vi "ROI_Selection_Limit.vi"(8 "error in (no error)":errorcluster, 9 "ROI in":T1, 10 "Square":bool, 11 "Picture":i32[][](array[numeric])) -> (0 "error out":errorcluster, 1 "ROI out":T1)   [LabVIEW 2011]
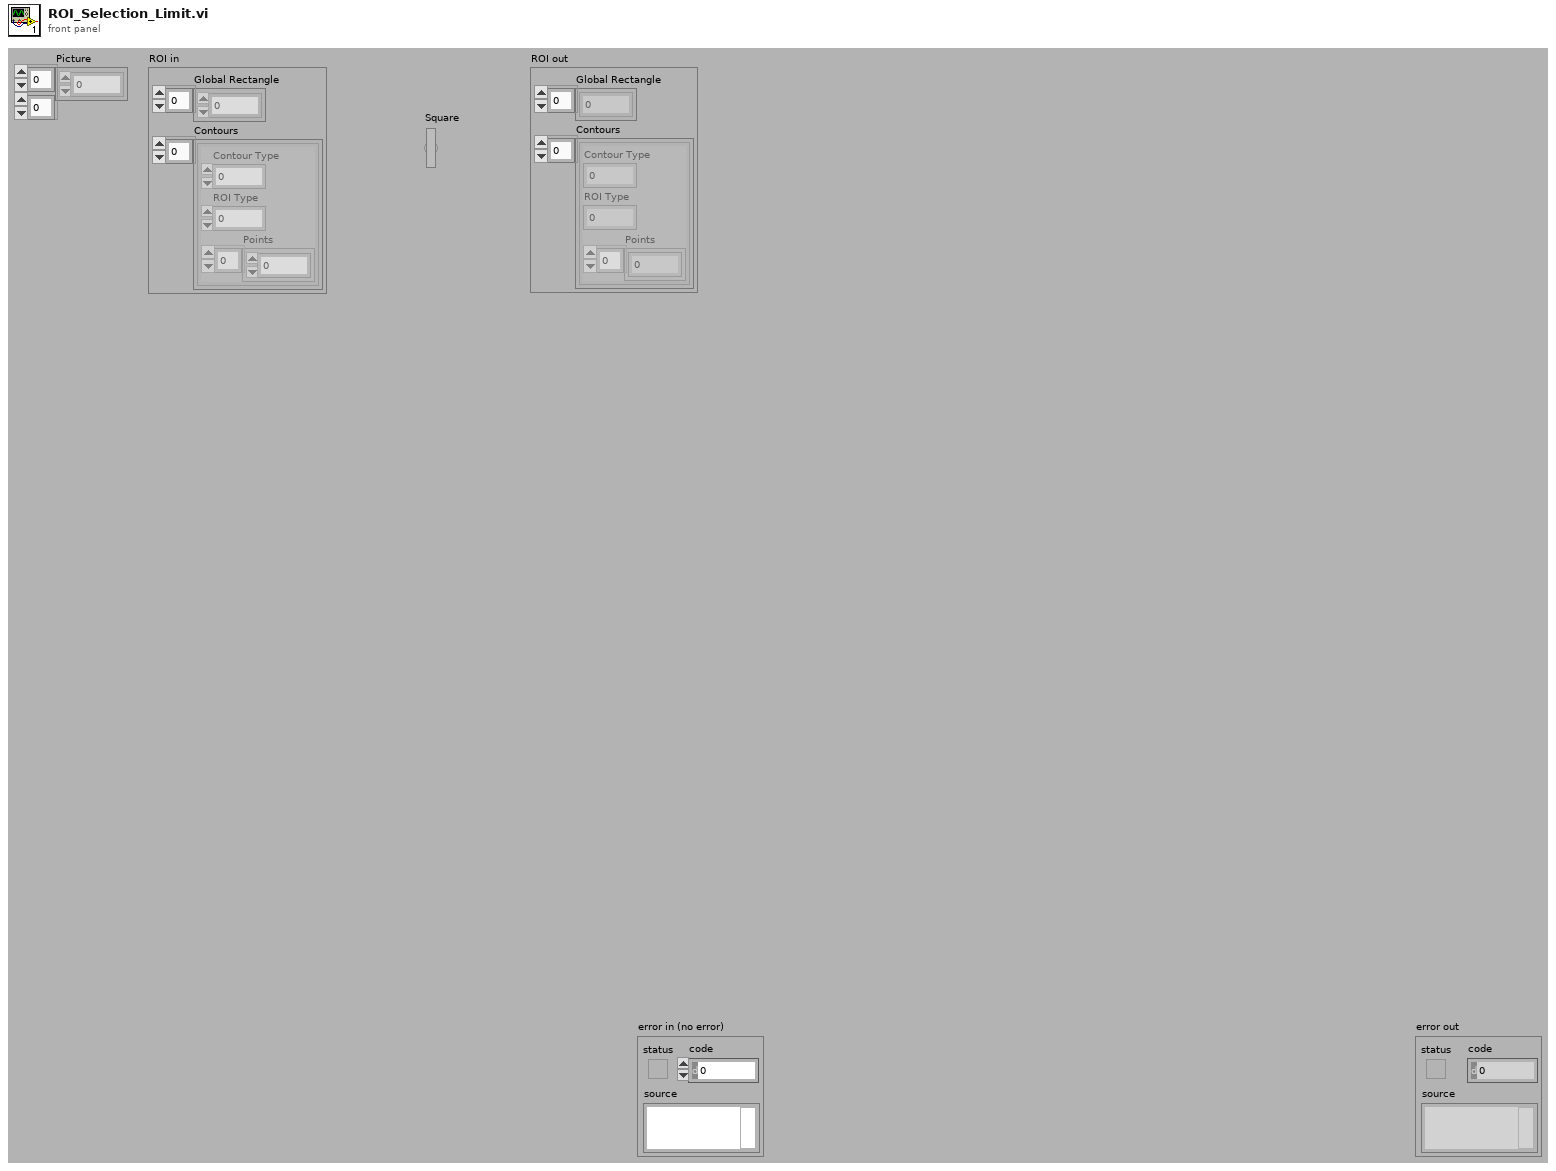
[diagram p1: front panel]
types:
  T1 = cluster{"Global Rectangle":i32[], "Contours":cluster{"Contour Type":u32, "ROI Type":u32, "Points":i32[]}[]}
  T2 = cluster{"Contour Type":u32, "ROI Type":u32, "Points":i32[]}[]
  T3 = cluster{"Contour Type":u32, "ROI Type":u32, "Points":i32[]}
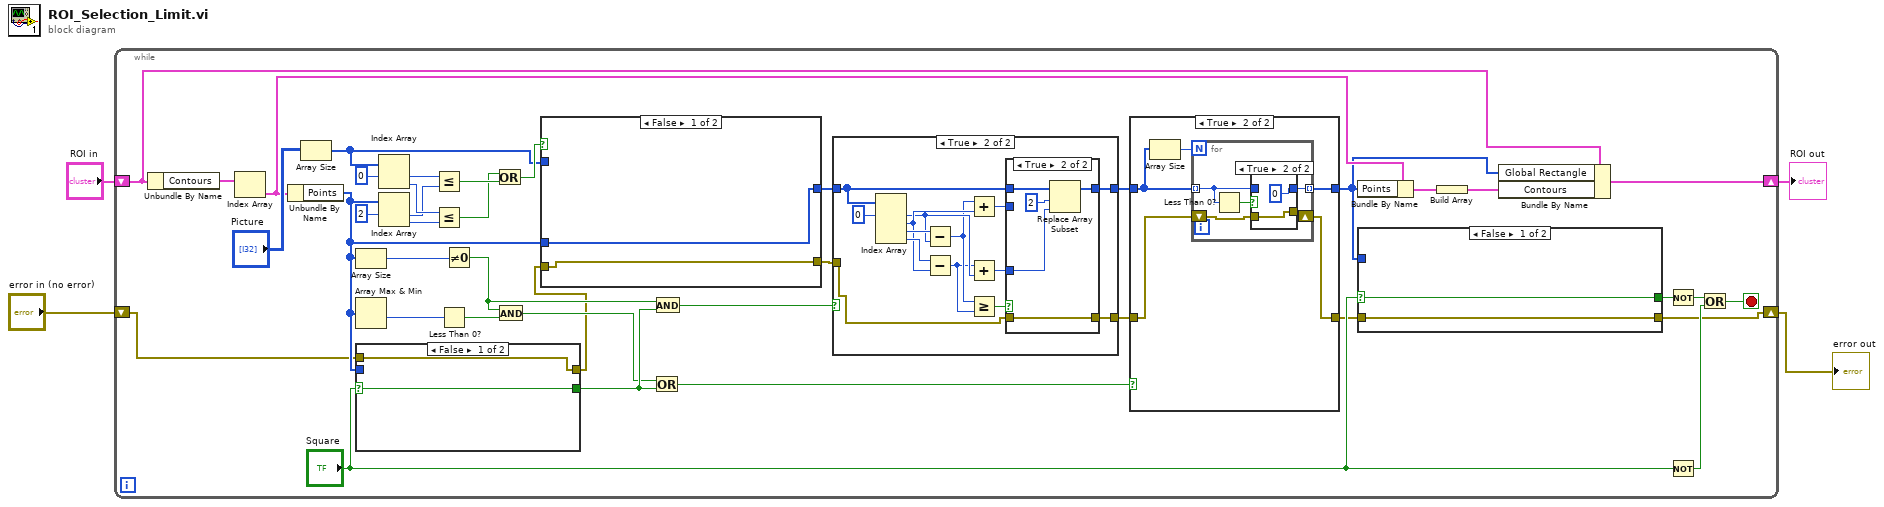
[diagram p0: block diagram]
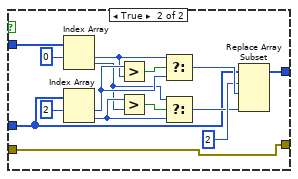
[diagram p2: hidden frame]
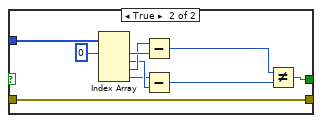
[diagram p3: hidden frame]
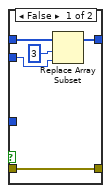
[diagram p5: hidden frame]
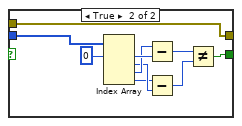
[diagram p6: hidden frame]
diagram:
  n1 = while {
    shift-right: [w27] -> w3
    shift-left: "ROI in" -> [w44]
    shift-right: [w10] -> w1
    shift-left: "error in (no error)" -> [w5]
    stop <- w26 stop-if-true
    n2 = Unbundle By Name(w44) -> ("Contours"=w22:T2)
    n3 = Index Array(array=w22) -> (element=w21:T3)  [unwired: 1 in]
    n4 = Unbundle By Name(w21) -> ("Points"=w13:i32[])
    n5 = Array Size(array="Picture") -> (size(s)=w11:i32[])
    n6 = Array Size(array=w13) -> (size(s)=w33:i32)
    n7 = Array Max & Min(array=w13) -> (min value=w32:i32)  [unwired: 3 out]
    n8 = case shown="False" "Square" {
      selector: "Square" -> [w101 _]
      tunnel: w13 -> [_ w111]
      tunnel: [w101 w103] -> w23
      tunnel: [w100 w102] -> w6
      tunnel: w5 -> [w100 w102]
      frame False {
      }
      frame True {
        n9 = Index Array(array=w111, index #1=0 ("index")) -> (element #1=w107:i32, element #2=w105:i32, element #3=w106:i32, element #4=w104:i32)  [unwired: 3 in]
        n10 = Subtract(x=w106, y=w107) -> (x-y=w109:i32)
        n11 = Subtract(x=w104, y=w105) -> (x-y=w108:i32)
        n12 = Not Equal?(x=w109, y=w108) -> (x != y?=w103:bool)
      }
    }
    n13 = Index Array(array=w11, index #1=0 ("index")) -> (element #1=w41:i32, element #2=w42:i32)  [unwired: 1 in]
    n14 = Index Array(array=w13, index #1=2 ("index")) -> (element #1=w36:i32, element #2=w37:i32)  [unwired: 1 in]
    n15 = Less Or Equal?(x=w41, y=w36) -> (x <= y?=w39:bool)
    n16 = Less Or Equal?(x=w42, y=w37) -> (x <= y?=w38:bool)
    n17 = Less Than 0?(x=w32) -> (x < 0?=w34:bool)
    n18 = Not Equal To 0?(x=w33) -> (x != 0?=w28:bool)
    n19 = Or(x=w38, y=w39) -> (x .or. y?=w14:bool)
    n20 = And(x=w28, y=w34) -> (x .and. y?=w15:bool)
    n21 = case shown="False" w14 {
      tunnel: w13 -> [w46 w50]
      tunnel: [w46 w48] -> w12
      tunnel: w11 -> [_ w49]
      tunnel: [w45 w47] -> w7
      tunnel: w6 -> [w45 w47]
      frame False {
      }
      frame True {
        n22 = Index Array(array=w49, index #1=0 ("index")) -> (element #1=w52:i32, element #2=w51:i32)  [unwired: 1 in]
        n23 = Index Array(array=w50, index #1=2 ("index")) -> (element #1=w59:i32, element #2=w57:i32)  [unwired: 1 in]
        n24 = Greater?(x=w59, y=w52) -> (0:w60:bool)
        n25 = Greater?(x=w57, y=w51) -> (0:w58:bool)
        n26 = Select(t=w52, s=w60, f=w59) -> (s? t:f=w56:i32)
        n27 = Select(t=w51, s=w58, f=w57) -> (s? t:f=w54:i32)
        n28 = Replace Array Subset(array=w50, new element #1=w56, index #1=2 ("index"), new element #2=w54) -> (w48:i32[])  [unwired: 1 in]
      }
    }
    n29 = Or(x=w15, y=w23) -> (x .or. y?=w31:bool)
    n30 = And(x=w28, y=w23) -> (x .and. y?=w30:bool)
    n31 = case shown="True" w30 {
      tunnel: [w75 w87] -> w29
      tunnel: w12 -> [w75 w78]
      tunnel: [w74 w77] -> w8
      tunnel: w7 -> [w74 w76]
      frame False {
      }
      frame True {
        n32 = Index Array(array=w78, index #1=0 ("index")) -> (element #1=w83:i32, element #2=w84:i32, element #3=w88:i32, element #4=w85:i32)  [unwired: 3 in]
        n33 = Subtract(x=w88, y=w83) -> (x-y=w82:i32)
        n34 = Subtract(x=w85, y=w84) -> (x-y=w81:i32)
        n35 = Add(x=w82, y=w84) -> (x+y=w86:i32)
        n36 = Add(x=w81, y=w83) -> (x+y=w79:i32)
        n37 = Greater Or Equal?(x=w82, y=w81) -> (x >= y?=w80:bool)
        n38 = case shown="True" w80 {
          tunnel: w78 -> [w94 w98]
          tunnel: [w93 w97] -> w87
          tunnel: w86 -> [w92 _]
          tunnel: w79 -> [_ w96]
          tunnel: w76 -> [w90 w95]
          tunnel: [w90 w95] -> w77
          frame False {
            n39 = Replace Array Subset(array=w94, new element=w92, index=3) -> (w93:i32[])
          }
          frame True {
            n40 = Replace Array Subset(array=w98, new element=w96, index=2) -> (w97:i32[])
          }
        }
      }
    }
    n41 = case shown="True" w31 {
      tunnel: w29 -> [w113 w117]
      tunnel: [w113 w116] -> w18
      tunnel: [w112 w114] -> w9
      tunnel: w8 -> [w112 w115]
      frame False {
      }
      frame True {
        n42 = Array Size(array=w117) -> (size(s)=w118:i32)
        n43 = for {
          N: w118 -> [_]
          tunnel: w117 -> [w122] mode=indexing
          tunnel: [w121] -> w116 mode=indexing
          shift-right: [w119] -> w114
          shift-left: w115 -> [w120]
          n44 = Less Than 0?(x=w122) -> (x < 0?=w123:bool)
          n45 = case shown="True" w123 {
            tunnel: w122 -> [w125 _]
            tunnel: [w125 0] -> w121
            tunnel: w120 -> [w124 w126]
            tunnel: [w124 w126] -> w119
            frame False {
            }
            frame True {
            }
          }
        }
      }
    }
    n46 = Bundle By Name(cluster=w21, "Points"=w18) -> (w20:T3)
    n47 = case shown="False" "Square" {
      selector: "Square" -> [w63 _]
      tunnel: w18 -> [_ w73]
      tunnel: [w63 w65] -> w16
      tunnel: [w62 w64] -> w10
      tunnel: w9 -> [w62 w64]
      frame False {
      }
      frame True {
        n48 = Index Array(array=w73, index #1=0 ("index")) -> (element #1=w69:i32, element #2=w67:i32, element #3=w68:i32, element #4=w66:i32)  [unwired: 3 in]
        n49 = Subtract(x=w68, y=w69) -> (x-y=w71:i32)
        n50 = Subtract(x=w66, y=w67) -> (x-y=w70:i32)
        n51 = Not Equal?(x=w71, y=w70) -> (x != y?=w65:bool)
      }
    }
    n52 = Build Array(w20) -> (w19:T2)
    n53 = Bundle By Name(cluster=w44, "Global Rectangle"=w18, "Contours"=w19) -> (w27:T1)
    n54 = Not(x=w16) -> (.not. x?=w24:bool)
    n55 = Not(x="Square") -> (.not. x?=w25:bool)
    n56 = Or(x=w24, y=w25) -> (x .or. y?=w26:bool)
  }
  "ROI out" <- w3
  "error out" <- w1
